vi "Dispose DataSet.vi"(8 "error in (no error)":errorcluster caption="错误输入（无错误）", 11 "DataSet 输入":refnum<class "DataSet.lvclass"> caption="DNL_LabVIEW Object in") -> (0 "error out":errorcluster caption="错误输出", 3 "DataSet 输出":refnum<class "DataSet.lvclass"> caption="DNL_LabVIEW Object out")   [LabVIEW 2012, in "Data Grid VIEW.lvlib" / "DataSet.lvclass"]
uses:
  DataSet.lvclass
  DataSet.lvclass/DataSet.ctl
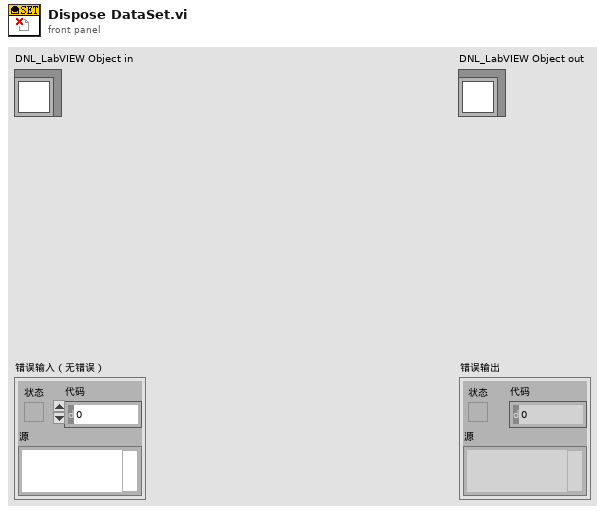
[diagram p1: front panel]
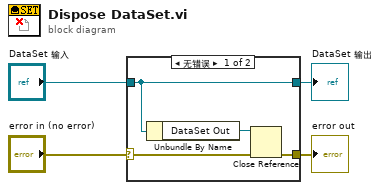
[diagram p0: block diagram]
diagram:
  n1 = case shown="无错误" "error in (no error)" {
    selector: "error in (no error)" -> [w6 w10]
    tunnel: [w5 w10] -> w3
    tunnel: [w8 w9] -> w1
    tunnel: "DataSet 输入" -> [w8 w9]
    frame No Error {
      n2 = Unbundle By Name(w8) -> ("DataSet Out"=w7:refnum<k24>)
      n3 = Close Reference(reference=w7, error in (no error)=w6) -> (error out=w5:errorcluster)
    }
    frame Error {
    }
  }
  "error out" <- w3
  "DataSet 输出" <- w1
